vi "zero.vi"() -> (3 "PositionOut":i32)   [LabVIEW 2014]
panel:
  in  "stop":bool
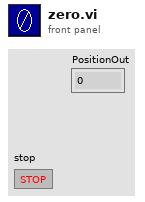
[diagram p1: front panel]
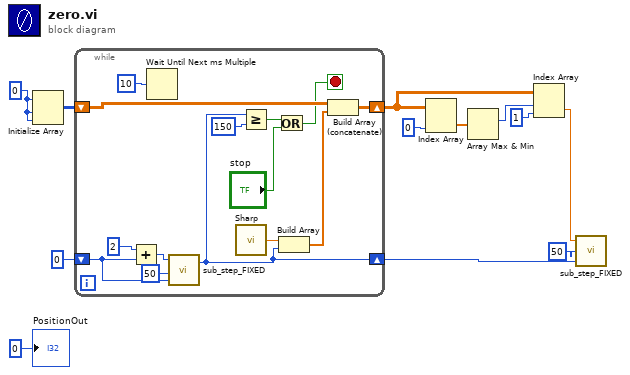
[diagram p0: block diagram]
diagram:
  w10 = 0
  n1 = Initialize Array(w10, w10, w10) -> (w11:i32[][])
  n2 = while {
    shift-right: [w16] -> w3
    shift-left: 0 -> [w24]
    shift-right: [w21] -> w6
    shift-left: w11 -> [w22]
    stop <- w18 stop-if-true
    n3 = Add(x=2, y=w24) -> (x+y=w25:i32)
    n4 = Wait Until Next ms Multiple(millisecond multiple=10) -> ()  [unwired: 1 out]
    n5 = call "sub_step_FIXED.vi"("Current Position"=w24, "millisecond multiple"=u32 50, "Desired Position"=w25) -> ("Position Out"=w16:i32)  [unwired: 1 in]
    n6 = call "Sharp.vi"() -> ("Slide 2"=w19:dbl)
    n7 = Greater Or Equal?(x=w16, y=150) -> (x >= y?=w15:bool)
    n8 = Or(x=w15, y="stop") -> (x .or. y?=w18:bool)
    n9 = Build Array(w19, w16) -> (w20:dbl[])
    n10 = Build Array (concatenate)(w22, w20) -> (w21:dbl[][])
  }
  n11 = Index Array(array=w6, index (col)=0) -> (element=w8:dbl[])  [unwired: 1 in]
  n12 = Array Max & Min(array=w8) -> (max index (indices)=w7:i32)  [unwired: 3 out]
  n13 = Index Array(array=w6, index (row)=w7, index (col)=1) -> (element=w4:dbl)
  n14 = call "sub_step_FIXED.vi"("Current Position"=w3, "millisecond multiple"=u32 50, "Desired Position"=w4) -> ()  [unwired: 1 in, 1 out]
  "PositionOut" <- 0
